vi "Check Device Status.vi"(8 "error in (no error)":errorcluster, 10 "Device GUID":string, 11 "Controller in":refnum<class "Controller.lvclass">) -> (0 "error out":errorcluster, 2 "Available?":bool, 3 "Controller out":refnum<class "Controller.lvclass">)   [LabVIEW 2016, in "Controller Actor.lvlib" / "Controller.lvclass"]
uses:
  <userlib>/Common Components/Controller/Controller.lvclass
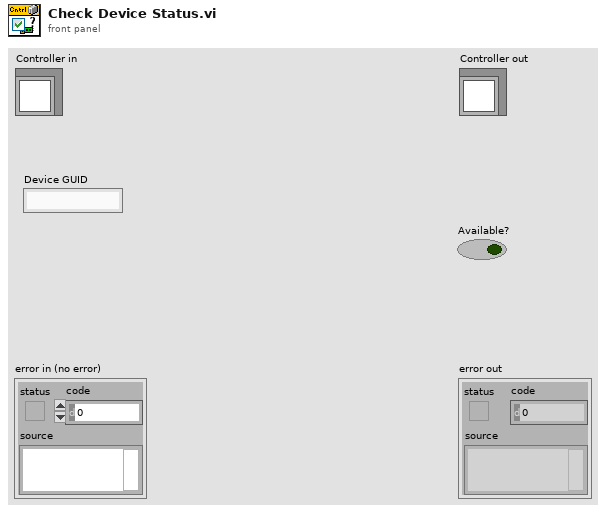
[diagram p1: front panel]
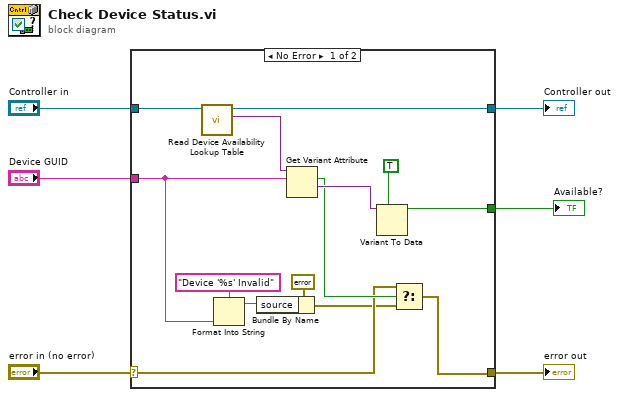
[diagram p0: block diagram]
diagram:
  n1 = case shown="No Error" "error in (no error)" {
    selector: "error in (no error)" -> [w13 w22]
    tunnel: [w12 w22] -> w5
    tunnel: [w19 w21] -> w3
    tunnel: "Controller in" -> [w20 w21]
    tunnel: "Device GUID" -> [w10 _]
    tunnel: [w16 _] -> w1
    frame No Error {
      n2 = call <userlib>:"Read Device Availability Lookup Table.vi"("Controller in"=w20) -> ("Device Availability Lookup Table"=w18:variant, "Controller out"=w19:refnum<class "Controller.lvclass">)  [unwired: 8 in, 1 out]
      n3 = Format Into String(format string="Device '%s' Invalid" ("source"), w10) -> (resulting string=w9:string)  [unwired: 2 in, 1 out]
      n4 = Bundle By Name(cluster=errorcluster {"status"=TRUE, "code"=5555, "source"="Device '%s' Invalid"} ("error constant"), "source"=w9) -> (w7:errorcluster)
      n5 = Get Variant Attribute(Variant=w18, name=w10) -> (found=w14:bool, value=w17:variant)  [unwired: 2 in, 2 out]
      n6 = Variant To Data(type=TRUE ("Available?"), Variant=w17) -> (data=w16:bool)  [unwired: 1 in, 1 out]
      n7 = Select(t=w13, s=w14, f=w7) -> (s? t:f=w12:errorcluster)
    }
    frame Error {
    }
  }
  "error out" <- w5
  "Controller out" <- w3
  "Available?" <- w1
